vi "GetParams.vi"(4 "Trans Geometry in":T1 {"focus location" format="%.2f"; "a (cm)" format="%.2f"; "Radius (cm)" format="%.2f"}, 5 "Path":path) -> (0 "Trans Geometry":T1 {"focus location" format="%.2f"; "a (cm)" format="%.2f"; "Radius (cm)" format="%.2f"}, 1 "Variables":T2={"Number of rings"=1, "sound spd (cm/s)"=150000, "z span (cm)"=4.0, "z steps"=20, "y span (cm)"=0.01, "y steps"=50, "time step (s)"=1e-08, "z"=0.0, "y"=0.0, "ref delay"=0.0, "freq (MHz)"=4.71, "cycles"=300} {"freq (MHz)" format="%.2f"; "z span (cm)" format="%.2f"; "y" format="%.2f"; "ref delay" format="%.2f"; "y span (cm)" format="%.3f"; "z" format="%.2f"; "time step (s)" format="%.2e"})   [LabVIEW 2022 SP3]
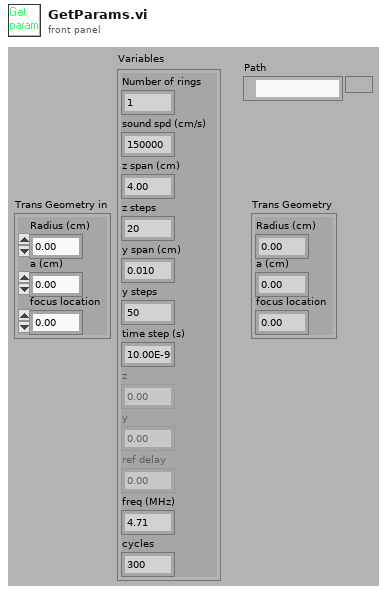
[diagram p1: front panel]
types:
  T1 = cluster{"Radius (cm)":dbl, "a (cm)":dbl, "focus location":dbl}
  T2 = cluster{"Number of rings":i32, "sound spd (cm/s)":i32, "z span (cm)":dbl, "z steps":i32, "y span (cm)":dbl, "y steps":i32, "time step (s)":sgl, "z":dbl, "y":dbl, "ref delay":dbl, "freq (MHz)":dbl, "cycles":i32}
  T3 = cluster{"Number of rings":i32, "sound spd (cm/s)":i32, "z span (cm)":dbl, "z steps":i32, "y spacing (cm)":dbl, "y steps":i32, "time step (s)":sgl, "z":dbl, "y":dbl, "ref delay":dbl, "y 2":dbl, "z steps 2":i32}
  T4 = cluster{"[0]":dbl, "[1]":dbl, "[2]":dbl, "[3]":dbl, "[4]":dbl, "[5]":dbl, "[6]":dbl, "[7]":dbl, "[8]":dbl}
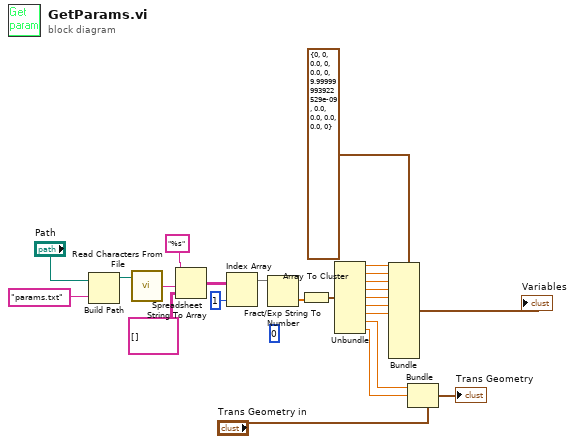
[diagram p0: block diagram]
diagram:
  (unwired) 0
  n1 = Build Path(base path="Path", name or relative path="params.txt") -> (appended path=w7:path)
  n2 = call <vilib>:"Read Characters From File.vi"("file path (dialog if empty)"=w7) -> ("character string"=w8:string)  [unwired: 1 in, 7 out]
  n3 = Spreadsheet String To Array(format string="%s", spreadsheet string=w8, array type (2D Dbl)=string[][] [] ("Array Constant")) -> (array=w10:string[][])  [unwired: 1 out]
  n4 = Index Array(array=w10, index (col)=1) -> (element=w13:string[])  [unwired: 1 in]
  n5 = Fract/Exp String To Number(string=w13) -> (number=w14:dbl[])  [unwired: 4 out]
  n6 = Array To Cluster(array=w14) -> (cluster=w15:T4)
  n7 = Unbundle(w15) -> ("[0]"=w16:dbl, "[1]"=w17:dbl, "[2]"=w18:dbl, "[3]"=w19:dbl, "[4]"=w20:dbl, "[5]"=w21:dbl, "[6]"=w22:dbl, "[7]"=w23:dbl, "[8]"=w24:dbl)
  n8 = Bundle(cluster=T3 {"Number of rings"=0, "sound spd (cm/s)"=0, "z span (cm)"=0.0, "z steps"=0, "y spacing (cm)"=0.0, "y steps"=0, "time step (s)"=1e-08, "z"=0.0, "y"=0.0, "ref delay"=0.0, "y 2"=0.0, "z steps 2"=0} ("Variables"), "Number of rings"=w16, "sound spd (cm/s)"=w17, "z span (cm)"=w18, "z steps"=w19, "y spacing (cm)"=w20, "y steps"=w21, "time step (s)"=w22) -> (→"Variables":T3)  [unwired: 5 out]
  n9 = Bundle(cluster="Trans Geometry in", "Radius (cm)"=w23, "a (cm)"=w24) -> (→"Trans Geometry":T1)  [unwired: 1 out]
